vi "Anti Jam.vi"   [LabVIEW 2016]
uses:
  Robot Global Data.vi
types:
  T1 = typedef "WPI_MotorControlDeviceRef.ctl" = cluster{"DeviceStatus":errorcluster, "Type":T2, "PWM":cluster{"PWM Channel":T3, "DeadBand":T4}, "CAN":cluster{"Device Number":u8, "SetOutput VI Ref":variant, "GetOutput VI Ref":variant, "Enable VI Ref":variant, "Disable VI Ref":variant, "Data":variant}, "Invert":bool}
  T2 = typedef "WPI_MotorControlType.ctl" = enum16{"PWM", "CAN"}
  T3 = typedef "FPGA_DIOPWMChannel.ctl" = enum8{"PWM 0", "PWM 1", "PWM 2", "PWM 3", "PWM 4", "PWM 5", "PWM 6", "PWM 7", "PWM 8", "PWM 9", "PWM MXP 0", "PWM MXP 1", "PWM MXP 2", "PWM MXP 3", "PWM MXP 4", "PWM MXP 5", "PWM MXP 6", "PWM MXP 7", "PWM MXP 8", "PWM MXP 9", "Invalid"}
  T4 = typedef "WPI_PWMDeadband.ctl" = cluster{"Name":string, "maxPositivePwm":i32, "minPositivePwm":i32, "centerPwm":i32, "maxNegativePwm":i32, "minNegativePwm":i32, "angularRange":u16}
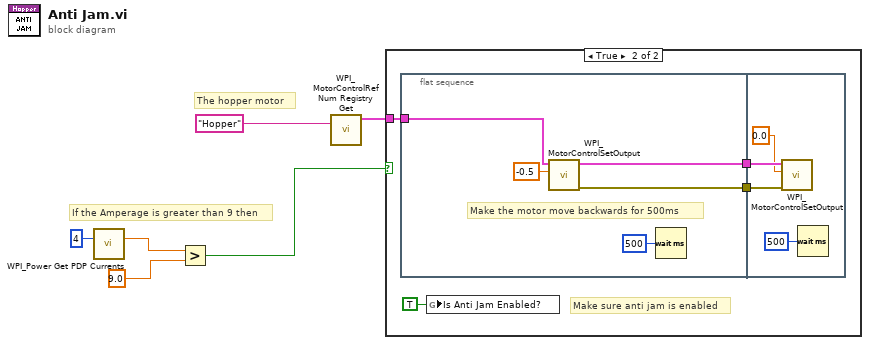
[diagram p0: block diagram]
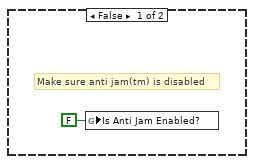
[diagram p2: hidden frame]
diagram:
  # "The hopper motor"
  # "If the Amperage is greater than 9 then"
  n1 = call <vilib>:"WPI_Power Get PDP Currents.vi"("PDP Channel"=4) -> ("current (A)"=w4:dbl)  [unwired: 12 in, 2 out]
  n2 = Greater?(x=w4, y=9.0) -> (0:w2:bool)
  n3 = call <vilib>:"WPI_MotorControlRefNum Registry Get.vi"("refnum name"="Hopper") -> ("MotorControlDevRef"=w3:T1)  [unwired: 9 in, 1 out]
  n4 = case shown="True" w2 {
    tunnel: w3 -> [_ w9]
    frame False {
      # "Make sure anti jam(tm) is disabled"
      n5 = global write "Robot Global Data.vi" "Is Anti Jam Enabled?"(FALSE ("Is Anti Jam Enabled?")) -> ()
    }
    frame True {
      # "Make sure anti jam is enabled"
      n6 = flat-sequence {
        tunnel: [w15] -> w11
        tunnel: [w14] -> w10
        tunnel: w9 -> [w12]
        tunnel: w11 -> [w19]
        tunnel: w10 -> [w18]
        frame #0 {
          # "Make the motor move backwards for 500ms"
          n7 = call <vilib>:"WPI_MotorControlSetOutput.vi"("Output"=-0.5, "MotorControlDevRef"=w12) -> ("error out"=w14:errorcluster, "MotorControlDevRef"=w15:T1)  [unwired: 7 in, 1 out]
          n8 = Wait (ms)(milliseconds to wait=u32 500) -> ()  [unwired: 1 out]
        }
        frame #1 {
          n9 = call <vilib>:"WPI_MotorControlSetOutput.vi"("error in (no error)"=w18, "Output"=0.0, "MotorControlDevRef"=w19) -> ()  [unwired: 6 in, 3 out]
          n10 = Wait (ms)(milliseconds to wait=u32 500) -> ()  [unwired: 1 out]
        }
      }
      n11 = global write "Robot Global Data.vi" "Is Anti Jam Enabled?"(TRUE ("Is Anti Jam Enabled?")) -> ()
    }
  }
